vi "Collect cantilever calibration metadata.vi"(0 "reference in":refnum<class "metadata.lvclass">, 5 "error in (no error)":errorcluster) -> (14 "reference out":refnum<class "metadata.lvclass">, 16 "Metadata":T1, 19 "error out":errorcluster)   [LabVIEW 2019, in "metadata.lvclass"]
uses:
  metadata.lvclass
  Metadata output --cluster.ctl
panel:
  out "List property names":string
  out "Property Names":string[](array[string])
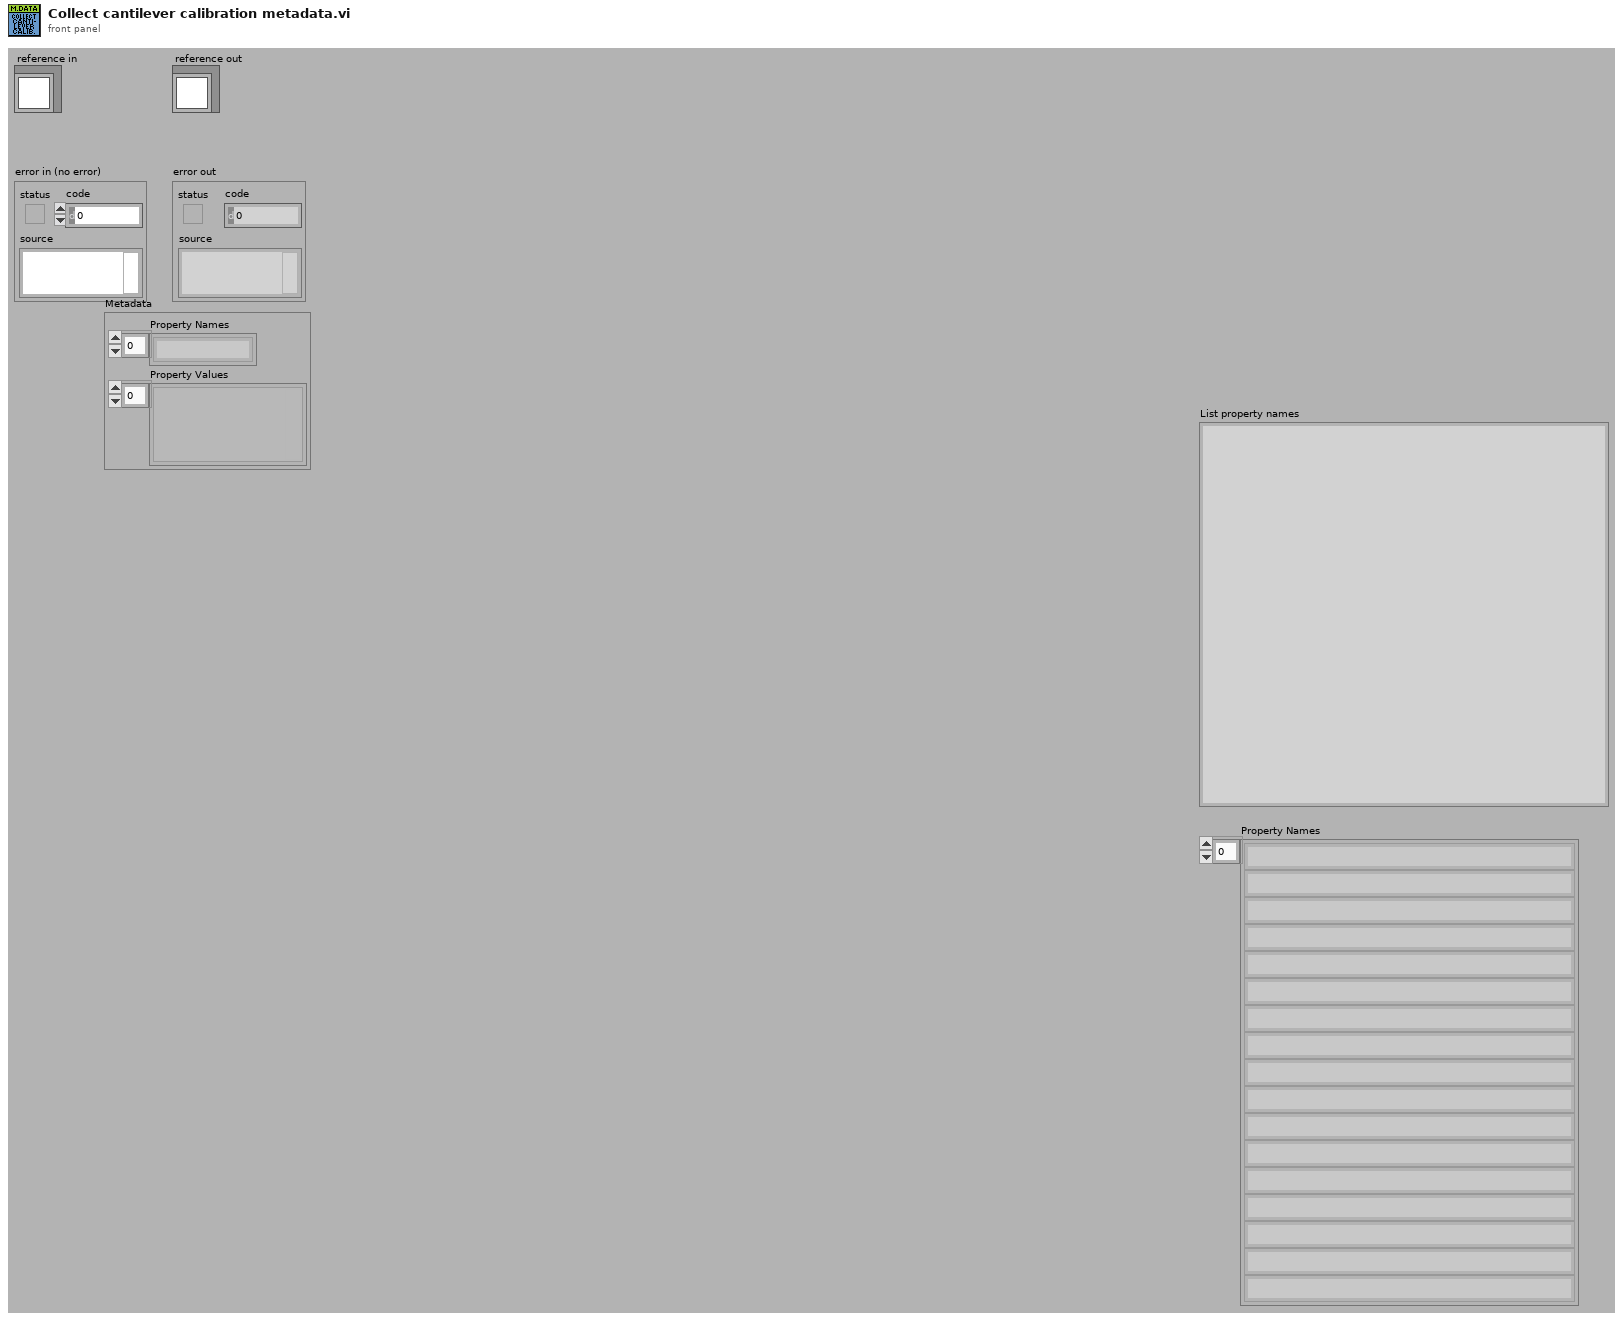
[diagram p1: front panel]
types:
  T1 = typedef "metadata.lvclass/Metadata output --cluster.ctl" = cluster{"Property Names":string[], "Property Values":variant[]}
  T2 = typedef "metadata.lvclass/ObjectAttributes.ctl" = cluster{"MyAttribute":dbl, "System Control":T3, "file info":T4, "Sample info":T5, "Cantilever info":T6, "XYZ piezos":T7, "Mapping":T8, "Fcurve segment":T9[], "Fast fpga segment":T11, "Chirp":T12, "precision (6)":i16, "width (-)":i16, "Metadata":T1, "config filepath":path, "Section names []":string[], "Property names []":string[], "nb elements":u16}
  T3 = typedef "metadata.lvclass/System control parameters.ctl" = cluster{"FPGA SW version":string, "TDMS file version":string, "Instrument":string, "Instrument model":string, "Instrument scanner":string, "Instrument clockrate (Mhz)":string, "Instrument tick time (us)":string}
  T4 = typedef "metadata.lvclass/File info parameters.ctl" = cluster{"Time Stamp":timestamp, "Filename":string, "Filepath":path, "User":string, "Experiment_name":string, "Curve_id":string, "number_segments":u8, "number_consecutive_scans":u32}
  T5 = typedef "metadata.lvclass/Sample info parameters.ctl" = cluster{"Sample name":string, "Sample species":string}
  T6 = typedef "metadata.lvclass/Cantilever info parameters.ctl" = cluster{"spring constant calib method":string, "invOLS calib method":string, "thermal calib deflection channel":string, "model":string, "shape":string, "tip geometry":string, "Laser sum (V)":dbl, "Laser power (mA)":dbl, "invOLS_(nm/V)":dbl, "spring constant nominal (N/m)":dbl, "spring constant calib (N/m)":dbl, "resosnance frequency air calib (Hz)":dbl, "resosnance frequency calib (Hz)":dbl, "quality factor":dbl, "Acoefficident_GCI_(nN.s^1.3/m)":dbl, "half angle (deg)":dbl, "tip radius (m)":dbl, "tip height (m)":dbl, "system mount angle (deg)":dbl}
  T7 = typedef "metadata.lvclass/XYZ piezos parameters.ctl" = cluster{"X stage piezo sensitivity (nm/V)":dbl, "X stage piezo gain":dbl, "X velocity (V/tick)":dbl, "X closed loop":bool, "Y stage piezo sensitivity (nm/V)":dbl, "Y stage piezo gain":dbl, "Y velocity (V/tick)":dbl, "Y closed loop":bool, "Z stage piezo sensitivity (nm/V)":dbl, "Z stage piezo gain":dbl, "Z closed loop":bool, "X position (V)":dbl, "Y position (V)":dbl}
  T8 = typedef "metadata.lvclass/Mapping parameters.ctl" = cluster{"Mapping":bool, "index":u16, "position row":u16, "position column":u16, "next position row":i16, "next position column":i16, "X initial position (V)":dbl, "Y initial position (V)":dbl, "X step size (V)":dbl, "Y step size (V)":dbl}
  T9 = typedef "metadata.lvclass/Fcurve segment.ctl" = cluster{"type":T10, "fast_fpga_trigger":bool, "nb":u8, "duration (ticks)":i64, "nb points":i32, "sampling rate (S/s)":u32, "Zpiezo control out":string, "initial deflection (V)":dbl, "relative setpoint":bool, "setpoint on":bool, "setpoint (V)":dbl, "setpoint trigger channel":string, "velocity (V/tick)":dbl, "Z position setpoint trigger (V)":dbl, "Z retract length (V)":dbl, "dec factor":u32}
  T10 = typedef "metadata.lvclass/Segment type--combobox.ctl" = string
  T11 = typedef "metadata.lvclass/fast fpga segment parameters.ctl" = cluster{"Fast start time trigger":timestamp, "nb_points":u32, "sampling_rate_(S/s)":u32, "duration_(ticks)":u32}
  T12 = typedef "metadata.lvclass/Chirp added parameters.ctl" = cluster{"f start (Hz)":dbl, "f end (Hz)":dbl, "Sweep type":string}
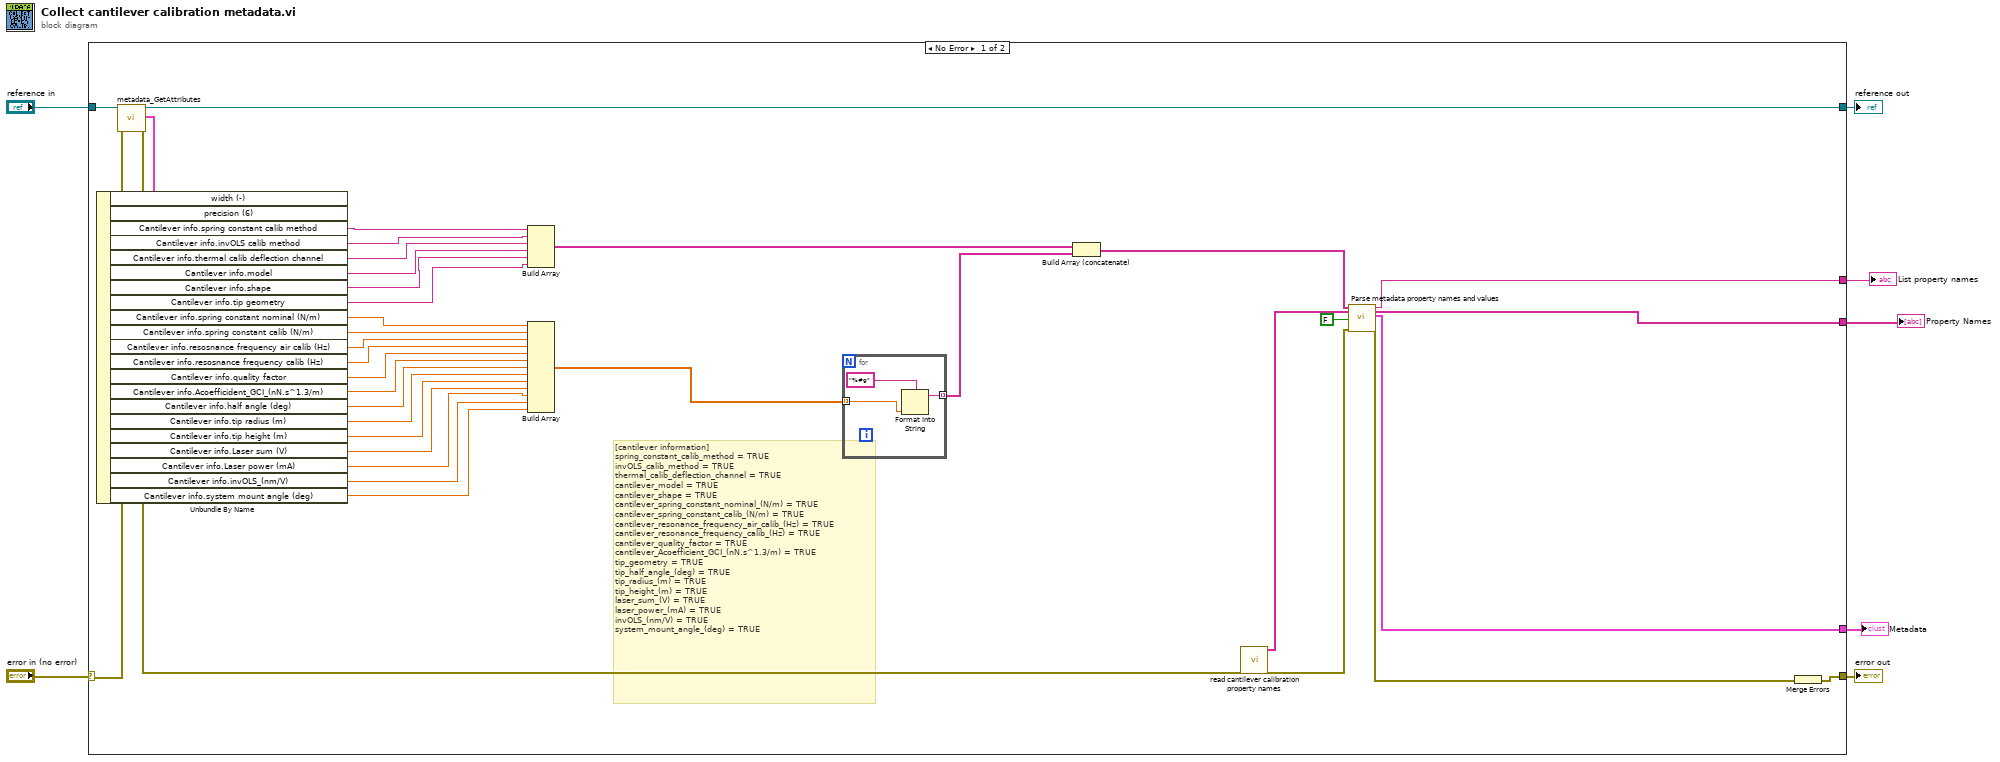
[diagram p0: block diagram]
diagram:
  n1 = case shown="No Error" "error in (no error)" {
    selector: "error in (no error)" -> [w40 w48]
    tunnel: [w43 w48] -> w6
    tunnel: [w41 w47] -> w4
    tunnel: "reference in" -> [w42 w47]
    tunnel: [w37 _] -> w3
    tunnel: [w36 _] -> w1
    tunnel: [w35 _] -> w2
    frame No Error {
      # "[cantilever information]\nspring_constant_calib_method = TRUE    \ninvOLS_calib_method = TRUE      \nthermal_calib_deflection_channel = TRUE      \ncantilever_model = TRUE    \ncantilever_shape = TRUE    \ncantilever_spring_constant_nominal_(N/m) = TRUE    \ncantilever_spring_constant_calib_(N/m) = TRUE    \ncantilever_resonance_frequency_air_calib_(Hz) = TRUE    \ncantilever_resonance_frequency_calib_(Hz) = TRUE    \ncantilever_quality_factor = TRUE    \ncantilever_Acoefficient_GCI_(nN.s^1.3/m) = TRUE    \ntip_geometry = TRUE    \ntip_half_angle_(deg) = TRUE    \ntip_radius_(m) = TRUE    \ntip_height_(m) = TRUE    \nlaser_sum_(V) = TRUE    \nlaser_power_(mA) = TRUE  \ninvOLS_(nm/V) = TRUE  \nsystem_mount_angle_(deg) = TRUE"
      n2 = call "metadata_GetAttributes.vi"("reference in"=w42, "error in (no error)"=w40) -> ("reference out"=w41:refnum<class "metadata.lvclass">, "attributes"=w39:T2, "error out"=w34:errorcluster)  [unwired: 14 in, 1 out]
      n3 = Unbundle By Name(w39) -> ("Cantilever info.spring constant calib method"=w19:string, "Cantilever info.invOLS calib method"=w18:string, "Cantilever info.thermal calib deflection channel"=w17:string, "Cantilever info.model"=w16:string, "Cantilever info.shape"=w15:string, "Cantilever info.tip geometry"=w14:string, "Cantilever info.spring constant nominal (N/m)"=w31:dbl, "Cantilever info.spring constant calib (N/m)"=w30:dbl, "Cantilever info.resosnance frequency air calib (Hz)"=w29:dbl, "Cantilever info.resosnance frequency calib (Hz)"=w28:dbl, "Cantilever info.quality factor"=w27:dbl, "Cantilever info.Acoefficident_GCI_(nN.s^1.3/m)"=w26:dbl, "Cantilever info.half angle (deg)"=w25:dbl, "Cantilever info.tip radius (m)"=w24:dbl, "Cantilever info.tip height (m)"=w23:dbl, "Cantilever info.Laser sum (V)"=w22:dbl, "Cantilever info.Laser power (mA)"=w21:dbl, "Cantilever info.invOLS_(nm/V)"=w20:dbl, "Cantilever info.system mount angle (deg)"=w8:dbl)  [unwired: 2 out]
      n4 = Build Array(w19, w18, w17, w16, w15, w14) -> (w13:string[])
      n5 = Build Array(w31, w30, w29, w28, w27, w26, w25, w24, w23, w22, w21, w20, w8) -> (w32:dbl[])
      n6 = for {
        tunnel: w32 -> [w44] mode=indexing
        tunnel: [w45] -> w12 mode=indexing
        n7 = Format Into String(format string="%#g", w44) -> (resulting string=w45:string)  [unwired: 2 in, 1 out]
      }
      n8 = Build Array (concatenate)(w13, w12) -> (w10:string[])
      n9 = call "read cantilever calibration property names.vi"("error in (no error)"=w34) -> ("Cantilever calib"=w11:string[], "error out"=w33:errorcluster)  [unwired: 17 in]
      n10 = call "Parse metadata property names and values.vi"("Data intput []"=w10, "property names []"=w11, "List param"=FALSE, "error in (no error)"=w33) -> ("Param list"=w35:string, "Array"=w37:string[], "output cluster"=w36:T1, "error out"=w38:errorcluster)  [unwired: 12 in]
      n11 = Merge Errors(w38) -> (w43:errorcluster)
    }
    frame Error {
    }
  }
  "error out" <- w6
  "reference out" <- w4
  "Property Names" <- w3
  "List property names" <- w2
  "Metadata" <- w1
